vi "Example.getAll.vi"(8 "error in (no error)":errorcluster, 11 "ExampleInstrument in":refnum<class "Example.lvclass">) -> (0 "error out":errorcluster, 2 "getAll":T1, 3 "ExampleInstrument out":refnum<class "Example.lvclass">)   [LabVIEW 2019, in "Example.lvclass"]
uses:
  Example.lvclass
  Typedefs/Example.getAll--Cluster.ctl
  caf7fc02-a1f0-4077-bb00-48bdf0fcd3b8.vi
  caf7fc02-a1f0-4077-bb00-48bdf0fcd3b8.vi/02299ac3-6fff-48cb-a6a6-d7db1d99cb7c.vi
  caf7fc02-a1f0-4077-bb00-48bdf0fcd3b8.vi/02299ac3-6fff-48cb-a6a6-d7db1d99cb7c.vi/44421b53-cfa9-4aa2-9699-77bcbc30e873.vi
  caf7fc02-a1f0-4077-bb00-48bdf0fcd3b8.vi/02299ac3-6fff-48cb-a6a6-d7db1d99cb7c.vi/164f2565-5067-42af-93ca-db5fc66b3116.vi
  caf7fc02-a1f0-4077-bb00-48bdf0fcd3b8.vi/02299ac3-6fff-48cb-a6a6-d7db1d99cb7c.vi/164f2565-5067-42af-93ca-db5fc66b3116.vi/07ebc684-d44b-4648-bcb1-00b39c506f23.vi
  caf7fc02-a1f0-4077-bb00-48bdf0fcd3b8.vi/02299ac3-6fff-48cb-a6a6-d7db1d99cb7c.vi/164f2565-5067-42af-93ca-db5fc66b3116.vi/3a3796ba-86d1-4358-9042-0c52ea7b8548.vi
  SMOs/RemoteControl/API/Remote Client.vi
  <vilib>/JDP Science/JSONtext/JSON text to Variant.vi
  <vilib>/JDP Science/JSONtext/LVClass Serializer/JSONtext LVClass Serializer.lvclass
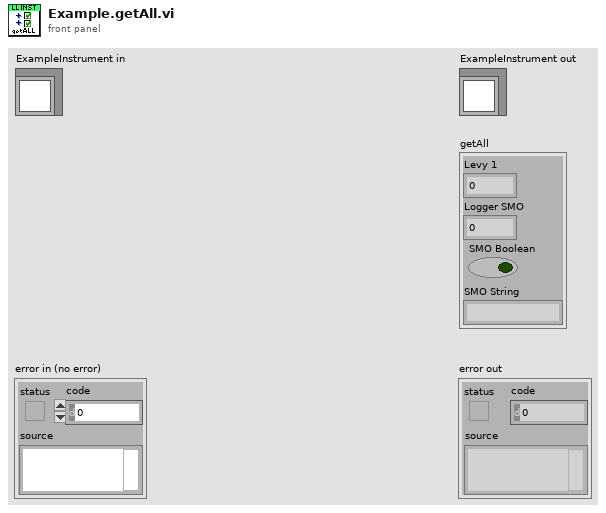
[diagram p1: front panel]
types:
  T1 = typedef "Example.lvclass/Example.getAll--Cluster.ctl" = cluster{"Levy 1":dbl, "Logger SMO":dbl, "SMO Boolean":bool, "SMO String":string}
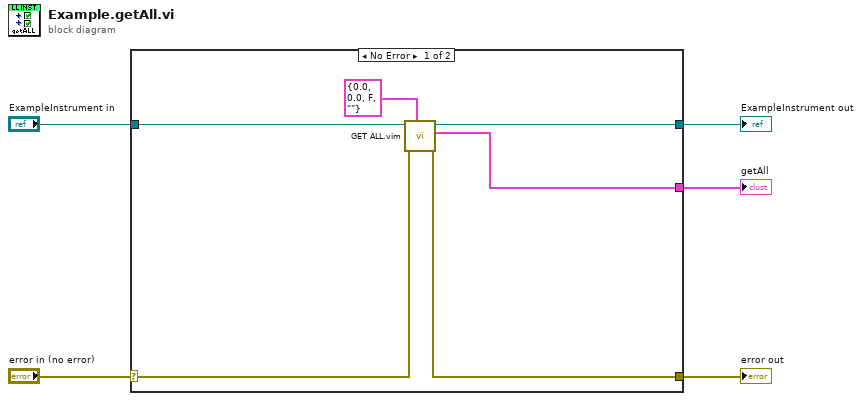
[diagram p0: block diagram]
diagram:
  n1 = case shown="No Error" "error in (no error)" {
    selector: "error in (no error)" -> [w9 w13]
    tunnel: [w8 w13] -> w4
    tunnel: [w10 w12] -> w2
    tunnel: "ExampleInstrument in" -> [w11 w12]
    tunnel: [w7 _] -> w1
    frame No Error {
      n2 = call "GET ALL.vim"("type"=T1 {"Levy 1"=0.0, "Logger SMO"=0.0, "SMO Boolean"=FALSE, "SMO String"=""} ("getAll"), "error in (no error)"=w9, "Instrument in"=w11) -> ("error out"=w8:errorcluster, "getAll"=w7:T1, "Instrument out"=w10:refnum<class "Example.lvclass">)  [unwired: 6 in]
    }
    frame Error {
    }
  }
  "error out" <- w4
  "ExampleInstrument out" <- w2
  "getAll" <- w1
